vi "myRIO_BRig_FPGA_resetOutputs_PortC.vi"   [LabVIEW 2014]
uses:
  <vilib>/rvi/eio/common/nirviEmuTemplateMethod_errors.vi
  <vilib>/eio/EIONode/EIONode.xnode
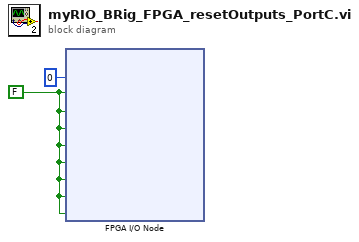
[diagram p0: block diagram]
diagram:
  w1 = FALSE ("ConnectorA/DIO3")
  n1 = xnode "FPGA I/O Node"("ConnectorC/AO0"=i16 0 ("ConnectorA/AO0"), "ConnectorC/DIO0"=w1, "ConnectorC/DIO1"=w1, "ConnectorC/DIO2"=w1, "ConnectorC/DIO3"=w1, "ConnectorC/DIO4"=w1, "ConnectorC/DIO5"=w1, "ConnectorC/DIO6"=w1, "ConnectorC/DIO7"=w1) -> ()  [unwired: 9 in, 9 out]
